vi "Core Geometry.vi"() -> (1 "Downcomer Gap (m)":dbl, 2 "Core Channel Equivalent Diameter (m)":dbl=0.1508, 3 "RX X-Section (m^2)":dbl)   [LabVIEW 2019]
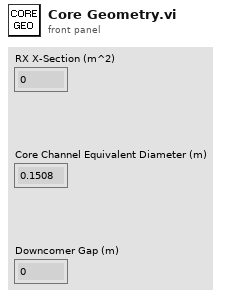
[diagram p1: front panel]
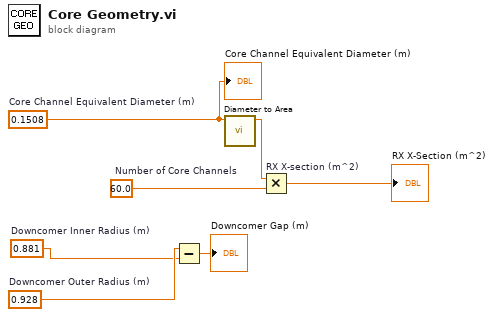
[diagram p0: block diagram]
diagram:
  w2 = 0.928  # Downcomer Outer Radius (m)
  w1 = 0.881  # Downcomer Inner Radius (m)
  w5 = 0.1508  # Core Channel Equivalent Diameter (m)
  w4 = 60.0  # Number of Core Channels
  n1 = Subtract(x=w2, y=w1) -> (x-y=→"Downcomer Gap (m)":dbl)
  n2 = call "Diameter to Area.vi"("Diameter (m)"=w5) -> ("Area (m^2)"=w6:dbl)  [unwired: 10 in]
  n3 = Multiply "RX X-section (m^2)"(x=w6, y=w4) -> (x*y=→"RX X-Section (m^2)":dbl)
  "Core Channel Equivalent Diameter (m)" <- w5
